vi "GTH-V2.Calibration.vi"(10 "Channel":enum16{"ChanA", "ChanB", "ChanC", "DAC"}(ring), 11 "VISA资源输入":refnum<visa-resource-name>="USB0::0x3323::0x0001::48E3845A3737::RAW") -> (0 "Error Out":errorcluster caption="错误输出", 3 "OK?":bool=TRUE)   [LabVIEW 2012, in "Lib_UEL.ATE.lvlib" / "STM32-CoreBD.lvlib"]
uses:
  STM32-CoreBD.lvlib
  <vilib>/Analysis/6fits.llb/Curve Fitting Criteria.ctl
  <vilib>/Utility/error.llb/whitespace.ctl
  <vilib>/Analysis/NI_AALPro.lvlib
panel:
  in  "Cal_DAC_Calibration":bool
  in  "Write_Data2GTH":bool
  out "Output":string[](array[string])=["\"2015-08-13,A10.032103,-65.663675\"", "\"2015-08-13,A20.012065,-24.682644\""]
  in  "Calibration Data":T1(array[cluster])=[{"ADC_Input"=1.0, "AD_Average"=5.0, "Code"="DAC"}, {"ADC_Input"=2.0, "AD_Average"=4.89, "Code"=""}, {"ADC_Input"=5.0, "AD_Average"=4.75, "Code"=""}, {"ADC_Input"=10.0, "AD_Average"=4.64, "Code"=""}, {"ADC_Input"=20.0, "AD_Average"=4.58, "Code"=""}, {"ADC_Input"=40.0, "AD_Average"=4.55, "Code"=""}, {"ADC_Input"=60.0, "AD_Average"=4.52, "Code"=""}]
  out "Best Linear Fit":dbl[][](array[numeric])=[[-3.0307985609221846, -3.030760037102811, -0.03999927599256473, -0.04186061853172174, 3.0287247066283762, 3.0301693498546984, -11.887892056086434, -11.886032639738248, 11.925863712026215, 11.928585419864591], [-3.009918735990917, -3.004162071768343, -0.02169820983103915, -0.021439537573563556, 3.0120375339021845, 3.005145559071942, -11.908703102077157, -11.899011096579235, 11.923308386282827, 11.920441274563307]] caption="最佳线性拟合"
  in  "Cal_ADC_Calibration":bool
  in  "停止":bool
  in  "RST_ADC_Value":bool
  in  "Get_ADC_Value":bool
  in  "ADC Input":dbl=11.914
  out "AD Average":dbl=3033.83968
  # "Version History\nV1.0.0, 2015-8-10, GTH-V2初始版本.\n- 每次使用前,请RST Calibration Data\n- ADC的数据是连接USB采样\n- CHAN A输入电压值: +/-3V, 0, +/-12V\n- CHAN B输入电压值: +/-1V, 0, +/-1.5V\n- CHAN C输入电压值: 1.xmA, 12.xmA\n\n- DAC数据需要手动输入.频率(Hz)幅度(mVpp)\n  1k,2k,5k,10k,20k,40k,60k\n   插上跳线帽,1k负载，1kHz，5VPP(1.76Vrms）"
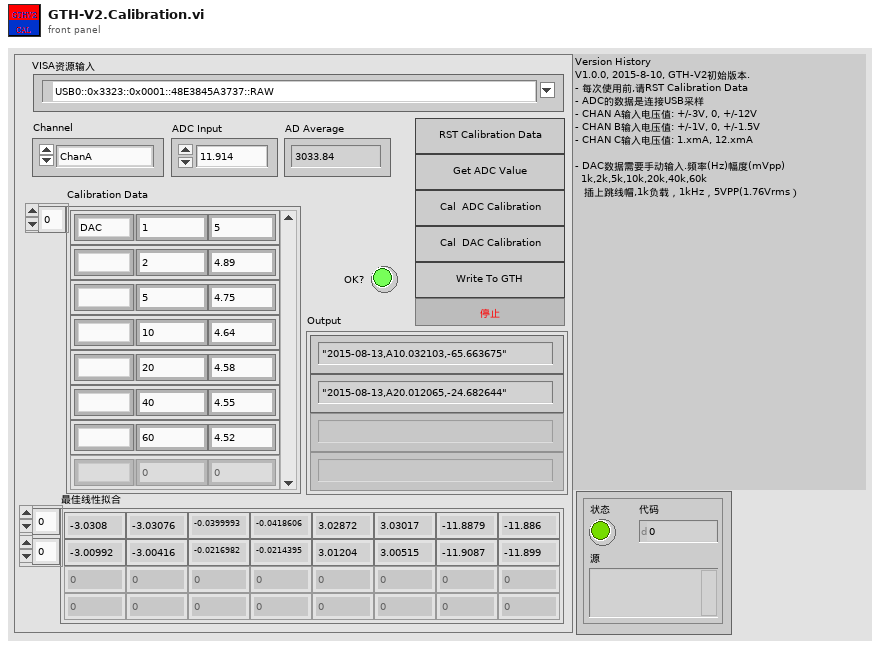
[diagram p1: front panel]
types:
  T1 = cluster{"ADC_Input":dbl, "AD_Average":dbl, "Code":string}[]
  T2 = enum16{"RelayA1", "RelayA2", "RelayA3", "RelayA4", "RelayA5", "RelayA6", "RelayA7", "RelayA8", "RelayA9", "RelayA10", "RelayB1", "RelayB2", "RelayB3", "RelayB4", "RelayB5", "RelayB6", "RelayB7", "RelayB8", "RelayB9", "RelayB10", "ADC1", "ADC2", "ADC3", "DAC1"}
  T3 = cluster{"ADC_Input":dbl, "AD_Average":dbl, "Code":string}
  T4 = enum16{"Read_Version", "Read_PID", "Read_CalibrationInfo", "Read_C_Value_ADC_ChanA", "Read_C_Value_ADC_ChanB", "Read_C_Value_Current", "Read_C_Value_DAC", "Write_CalibrationInfo", "Write_C_Value_ADC_ChanA", "Write_C_Value_ADC_ChanB", "Write_C_Value_Current", "Write_C_Value_DAC"}
  T5 = typedef "NI_AALPro.lvlib/Curve Fitting Criteria.ctl" = u16
  T6 = typedef "whitespace.ctl" = u16
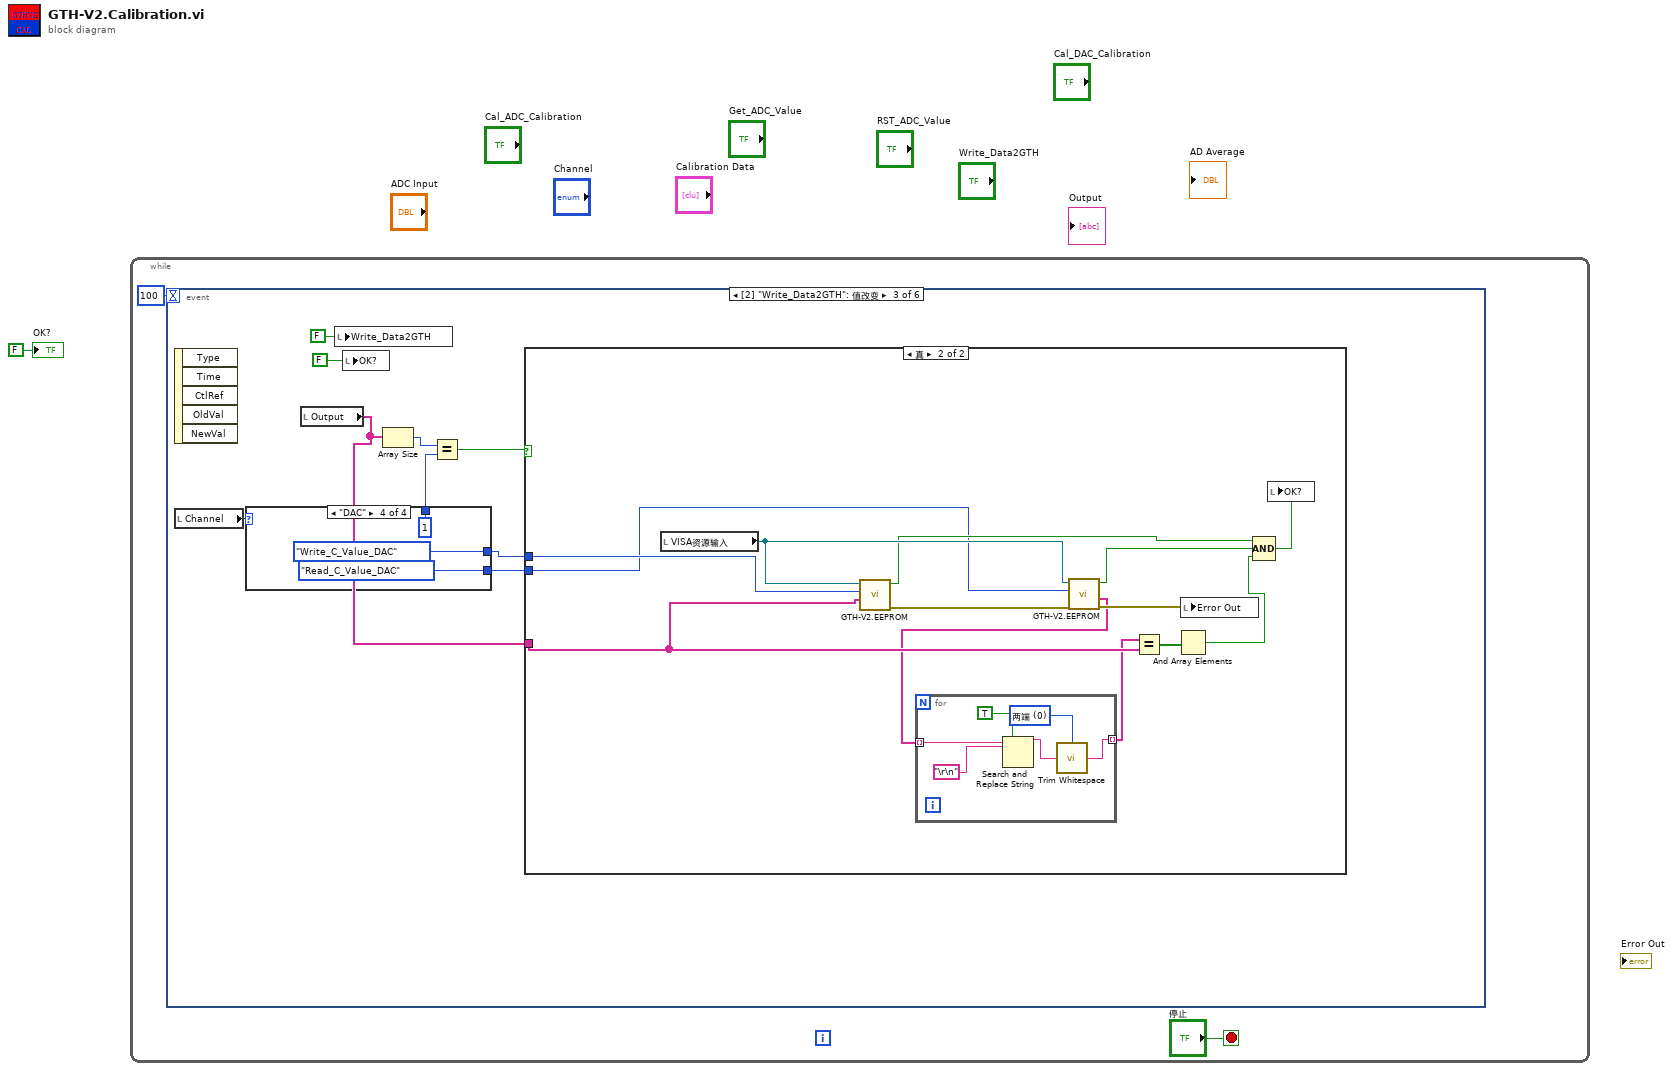
[diagram p0: block diagram]
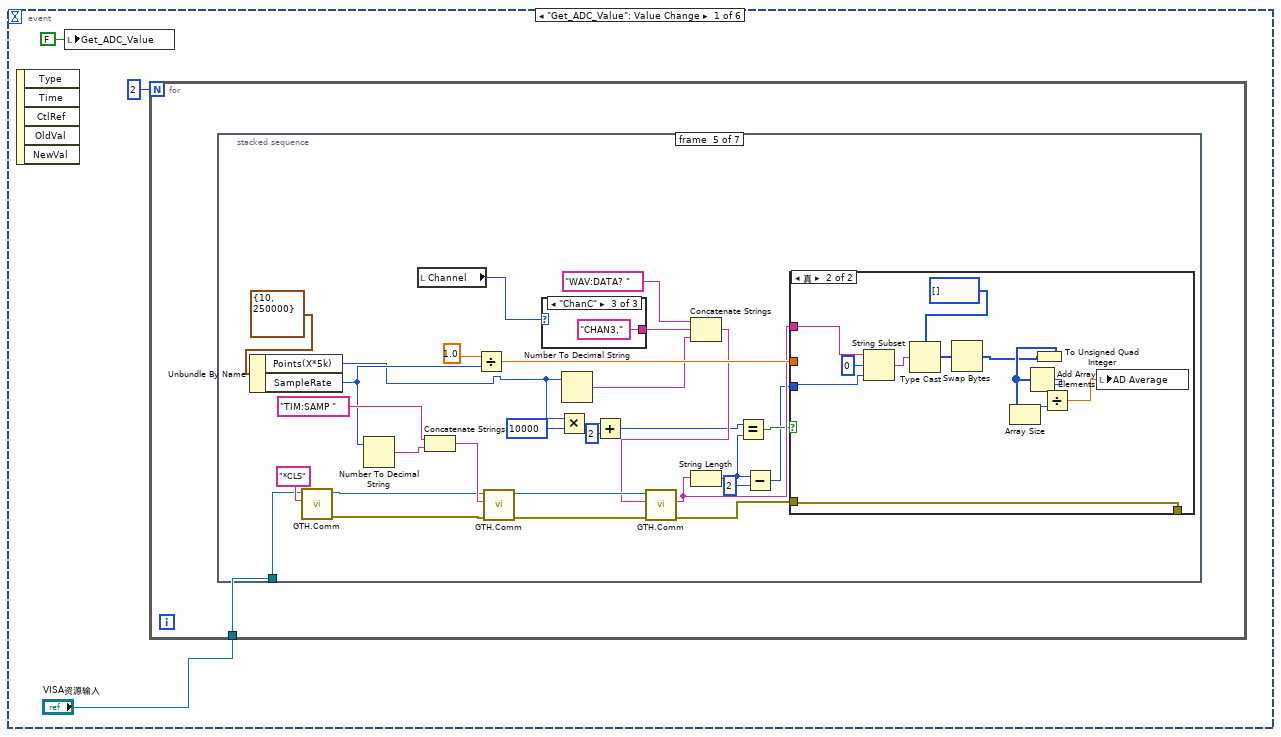
[diagram p2: hidden frame]
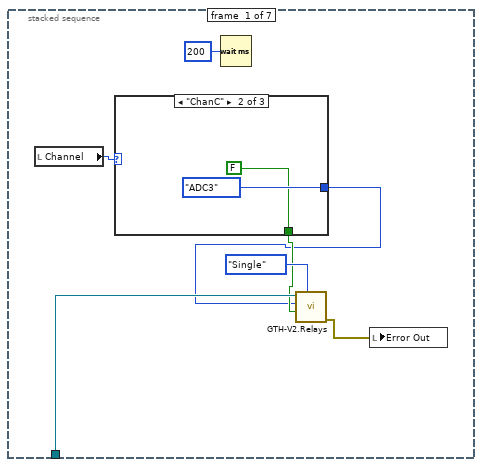
[diagram p3: hidden frame]
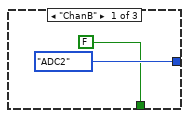
[diagram p4: hidden frame]
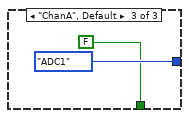
[diagram p5: hidden frame]
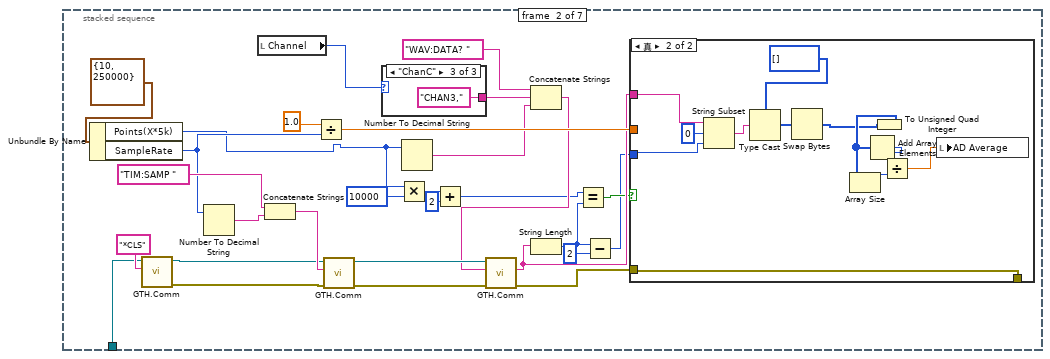
[diagram p6: hidden frame]
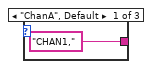
[diagram p8: hidden frame]
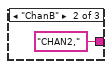
[diagram p9: hidden frame]
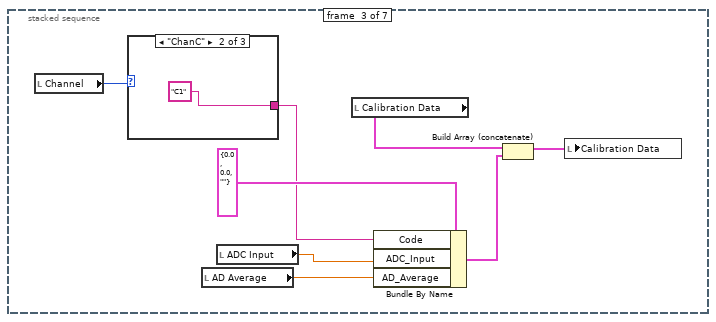
[diagram p10: hidden frame]
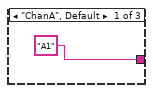
[diagram p11: hidden frame]
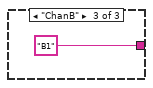
[diagram p12: hidden frame]
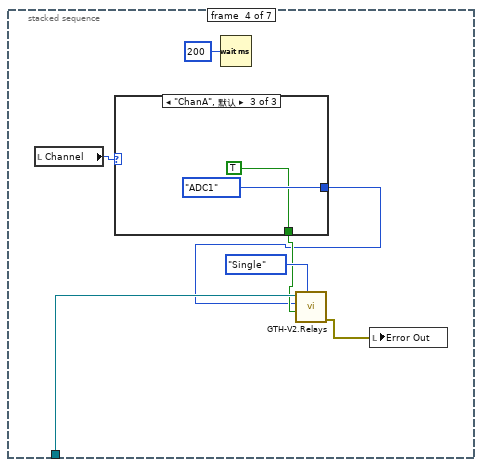
[diagram p13: hidden frame]
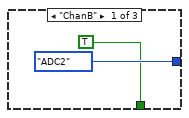
[diagram p14: hidden frame]
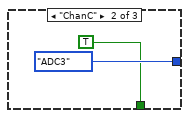
[diagram p15: hidden frame]
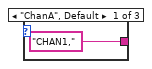
[diagram p17: hidden frame]
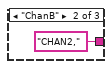
[diagram p18: hidden frame]
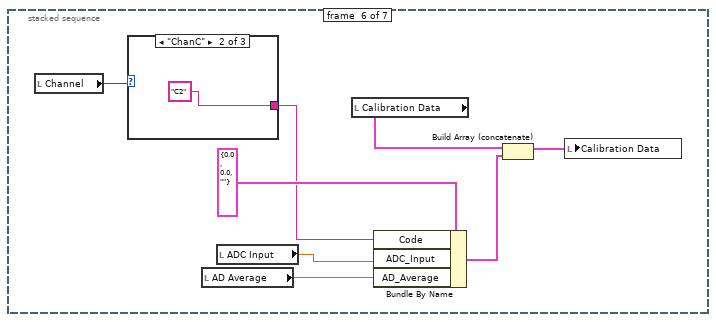
[diagram p19: hidden frame]
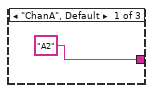
[diagram p20: hidden frame]
diagram:
  n1 = while {
    stop <- "停止" stop-if-true
    n2 = event shown="[2] \"Write_Data2GTH\": 值改变" {
      selector: _ -> [_ _ _ _ _ _]
      dyn-events: _ -> [_ _ _ _ _ _]
      timeout: 100 -> [_ _ _ _ _ _]
      event "Get_ADC_Value": Value Change {
        n3 = event-data() -> ()  [unwired: 1 in, 5 out]
        n4 = local write "Get_ADC_Value"(FALSE ("Get_ADC_Value")) -> ()
        n5 = for {
          N: 2 -> [_]
          tunnel: "VISA资源输入" -> [w7]
          n6 = stacked-sequence {
            tunnel: w7 -> [w12 w23 _ w81 w92 _ _]
            frame #0 {
              n7 = local read "Channel"() -> (w10:enum16{"ChanA", "ChanB", "ChanC", "DAC"})
              n8 = case shown="\"ChanC\"" w10 {
                tunnel: [T2."ADC2" ("Para") T2."ADC3" ("Para") T2."ADC1" ("Para")] -> w8
                tunnel: [FALSE ("ON/FF") FALSE ("ON/FF") FALSE ("ON/FF")] -> w9
                frame "ChanB" {
                }
                frame "ChanC" {
                }
                frame "ChanA", Default {
                }
              }
              n9 = Wait (ms)(milliseconds to wait=u32 200 ("等待时间（毫秒）")) -> ()  [unwired: 1 out]
              n10 = call "GTH-V2.Relays.vi"("CMD"=enum16{"All", "ChanA", "ChanB", "Single"}."Single", "ON/FF"=w9, "Para"=w8, "VISA资源输入"=w12) -> ("Error Out"=w13:errorcluster)  [unwired: 5 in, 2 out]
              n11 = local write "Error Out"(w13) -> ()
            }
            frame #1 {
              n12 = Unbundle By Name(cluster{"Points(X*5k)":u8, "SampleRate":u32} {"Points(X*5k)"=10, "SampleRate"=250000} ("ADC_Para")) -> ("Points(X*5k)"=w24:u8, "SampleRate"=w25:u32)
              n13 = call "GTH.Comm.vi"("SCPI CMD"="*CLS" ("字符串"), "USB Port In"=w23) -> ("Error Out"=w40:errorcluster, "USB Port Out"=w41:refnum<visa-resource-name>)  [unwired: 4 in, 4 out]
              n14 = Number To Decimal String(number=w25) -> (decimal integer string=w43:string)  [unwired: 1 in]
              n15 = local read "Channel"() -> (w21:enum16{"ChanA", "ChanB", "ChanC", "DAC"})
              n16 = Concatenate Strings("TIM:SAMP " ("字符串"), w43) -> (w42:string)
              n17 = Divide(x=1.0 ("y"), y=w25) -> (x/y=w46:dbl)
              n18 = call "GTH.Comm.vi"("Error In"=w40, "SCPI CMD"=w42, "USB Port In"=w41) -> ("Error Out"=w37:errorcluster, "USB Port Out"=w38:refnum<visa-resource-name>)  [unwired: 3 in, 4 out]
              n19 = case shown="\"ChanC\"" w21 {
                tunnel: ["CHAN1," ("字符串") "CHAN2," ("字符串") "CHAN3," ("字符串")] -> w48
                frame "ChanA", Default {
                }
                frame "ChanB" {
                }
                frame "ChanC" {
                }
              }
              n20 = Multiply(x=w24, y=u32 10000) -> (x*y=w33:u32)
              n21 = Number To Decimal String(number=w24) -> (decimal integer string=w39:string)  [unwired: 1 in]
              n22 = Add(x=w33, y=u32 2) -> (x+y=w30:u32)
              n23 = Concatenate Strings("WAV:DATA? " ("字符串"), w48, w39) -> (w36:string)
              n24 = call "GTH.Comm.vi"("Error In"=w37, "SCPI CMD"=w36, "USB Port In"=w38) -> ("Error Out"=w35:errorcluster, "Return"=w31:string)  [unwired: 3 in, 4 out]
              n25 = String Length(string=w31) -> (length=w28:i32)
              n26 = Equal?(x=w30, y=w28) -> (x = y?=w29:bool)
              n27 = Subtract(x=w28, y=2) -> (x-y=w26:i32)
              n28 = case shown="真" w29 {
                tunnel: w46 -> [_ _]
                tunnel: [w50 w52] -> _
                tunnel: w35 -> [w50 w52]
                tunnel: w31 -> [_ w59]
                tunnel: w26 -> [_ w57]
                frame False {
                }
                frame True {
                  n29 = String Subset(string=w59, offset (0)=0 ("偏移量(0)"), length (rest)=w57) -> (substring=w60:string)
                  n30 = Type Cast(type=u16[] [], x=w60) -> (*(type *) &x=w61:u16[])
                  n31 = Swap Bytes(anything=w61) -> (byte swapped=w53:u16[])
                  n32 = To Unsigned Quad Integer(1:w53) -> (0:w54:u64[])
                  n33 = Array Size(array=w54) -> (size(s)=w55:i32)
                  n34 = Add Array Elements(numeric array=w54) -> (sum=w56:u64)
                  n35 = Divide(x=w56, y=w55) -> (x/y=w51:dbl)
                  n36 = local write "AD Average"(w51) -> ()
                }
              }
            }
            frame #2 {
              n37 = local read "Channel"() -> (w66:enum16{"ChanA", "ChanB", "ChanC", "DAC"})
              n38 = case shown="\"ChanC\"" w66 {
                tunnel: ["A1" ("Code") "C1" ("Code") "B1" ("Code")] -> w67
                frame "ChanA", Default {
                }
                frame "ChanC" {
                }
                frame "ChanB" {
                }
              }
              n39 = local read "AD Average"() -> (w72:dbl)
              n40 = local read "ADC Input"() -> (w71:dbl)
              n41 = local read "Calibration Data"() -> (w70:T1)
              n42 = Bundle By Name(cluster=T3 {"ADC_Input"=0.0, "AD_Average"=0.0, "Code"=""} ("簇"), "Code"=w67, "ADC_Input"=w71, "AD_Average"=w72) -> (w69:T3)
              n43 = Build Array (concatenate)(w70, w69) -> (w68:T1)
              n44 = local write "Calibration Data"(w68) -> ()
            }
            frame #3 {
              n45 = local read "Channel"() -> (w79:enum16{"ChanA", "ChanB", "ChanC", "DAC"})
              n46 = case shown="\"ChanA\", 默认" w79 {
                tunnel: [T2."ADC2" ("Para") T2."ADC3" ("Para") T2."ADC1" ("Para")] -> w77
                tunnel: [TRUE ("ON/FF") TRUE ("ON/FF") TRUE ("ON/FF")] -> w78
                frame "ChanB" {
                }
                frame "ChanC" {
                }
                frame "ChanA", Default {
                }
              }
              n47 = Wait (ms)(milliseconds to wait=u32 200 ("等待时间（毫秒）")) -> ()  [unwired: 1 out]
              n48 = call "GTH-V2.Relays.vi"("CMD"=enum16{"All", "ChanA", "ChanB", "Single"}."Single", "ON/FF"=w78, "Para"=w77, "VISA资源输入"=w81) -> ("Error Out"=w82:errorcluster)  [unwired: 5 in, 2 out]
              n49 = local write "Error Out"(w82) -> ()
            }
            frame #4 {
              n50 = Unbundle By Name(cluster{"Points(X*5k)":u8, "SampleRate":u32} {"Points(X*5k)"=10, "SampleRate"=250000} ("ADC_Para")) -> ("Points(X*5k)"=w93:u8, "SampleRate"=w94:u32)
              n51 = call "GTH.Comm.vi"("SCPI CMD"="*CLS" ("字符串"), "USB Port In"=w92) -> ("Error Out"=w109:errorcluster, "USB Port Out"=w110:refnum<visa-resource-name>)  [unwired: 4 in, 4 out]
              n52 = Number To Decimal String(number=w94) -> (decimal integer string=w112:string)  [unwired: 1 in]
              n53 = local read "Channel"() -> (w90:enum16{"ChanA", "ChanB", "ChanC", "DAC"})
              n54 = Concatenate Strings("TIM:SAMP " ("字符串"), w112) -> (w111:string)
              n55 = Divide(x=1.0 ("y"), y=w94) -> (x/y=w115:dbl)
              n56 = call "GTH.Comm.vi"("Error In"=w109, "SCPI CMD"=w111, "USB Port In"=w110) -> ("Error Out"=w106:errorcluster, "USB Port Out"=w107:refnum<visa-resource-name>)  [unwired: 3 in, 4 out]
              n57 = case shown="\"ChanC\"" w90 {
                tunnel: ["CHAN1," ("字符串") "CHAN2," ("字符串") "CHAN3," ("字符串")] -> w117
                frame "ChanA", Default {
                }
                frame "ChanB" {
                }
                frame "ChanC" {
                }
              }
              n58 = Multiply(x=w93, y=u32 10000) -> (x*y=w102:u32)
              n59 = Number To Decimal String(number=w93) -> (decimal integer string=w108:string)  [unwired: 1 in]
              n60 = Add(x=w102, y=u32 2) -> (x+y=w99:u32)
              n61 = Concatenate Strings("WAV:DATA? " ("字符串"), w117, w108) -> (w105:string)
              n62 = call "GTH.Comm.vi"("Error In"=w106, "SCPI CMD"=w105, "USB Port In"=w107) -> ("Error Out"=w104:errorcluster, "Return"=w100:string)  [unwired: 3 in, 4 out]
              n63 = String Length(string=w100) -> (length=w97:i32)
              n64 = Equal?(x=w99, y=w97) -> (x = y?=w98:bool)
              n65 = Subtract(x=w97, y=2) -> (x-y=w95:i32)
              n66 = case shown="真" w98 {
                tunnel: w115 -> [_ _]
                tunnel: [w119 w121] -> _
                tunnel: w104 -> [w119 w121]
                tunnel: w100 -> [_ w128]
                tunnel: w95 -> [_ w126]
                frame False {
                }
                frame True {
                  n67 = String Subset(string=w128, offset (0)=0 ("偏移量(0)"), length (rest)=w126) -> (substring=w129:string)
                  n68 = Type Cast(type=u16[] [], x=w129) -> (*(type *) &x=w130:u16[])
                  n69 = Swap Bytes(anything=w130) -> (byte swapped=w122:u16[])
                  n70 = To Unsigned Quad Integer(1:w122) -> (0:w123:u64[])
                  n71 = Array Size(array=w123) -> (size(s)=w124:i32)
                  n72 = Add Array Elements(numeric array=w123) -> (sum=w125:u64)
                  n73 = Divide(x=w125, y=w124) -> (x/y=w120:dbl)
                  n74 = local write "AD Average"(w120) -> ()
                }
              }
            }
            frame #5 {
              n75 = local read "Channel"() -> (w135:enum16{"ChanA", "ChanB", "ChanC", "DAC"})
              n76 = case shown="\"ChanC\"" w135 {
                tunnel: ["A2" ("Code") "C2" ("Code") "B2" ("Code")] -> w136
                frame "ChanA", Default {
                }
                frame "ChanC" {
                }
                frame "ChanB" {
                }
              }
              n77 = local read "AD Average"() -> (w141:dbl)
              n78 = local read "ADC Input"() -> (w140:dbl)
              n79 = local read "Calibration Data"() -> (w139:T1)
              n80 = Bundle By Name(cluster=T3 {"ADC_Input"=0.0, "AD_Average"=0.0, "Code"=""} ("簇"), "Code"=w136, "ADC_Input"=w140, "AD_Average"=w141) -> (w138:T3)
              n81 = Build Array (concatenate)(w139, w138) -> (w137:T1)
              n82 = local write "Calibration Data"(w137) -> ()
            }
            frame #6 {
              n83 = Wait (ms)(milliseconds to wait=u32 500 ("等待时间（毫秒）")) -> ()  [unwired: 1 out]
            }
          }
        }
      }
      event "Cal_DAC_Calibration": Value Change {
        n84 = event-data() -> ()  [unwired: 1 in, 5 out]
        n85 = local read "Calibration Data"() -> (w150:T1)
        n86 = local write "Cal_DAC_Calibration"(FALSE ("Cal_DAC_Calibration")) -> ()
        n87 = Array Size(array=w150) -> (size(s)=w149:i32)
        n88 = Greater Or Equal?(x=w149, y=6) -> (x >= y?=w147:bool)
        n89 = case shown="真" w147 {
          tunnel: w150 -> [_ w170]
          frame False {
          }
          frame True {
            w160 = "," ("时间格式字符串(%c)")
            w169 = T5 0 items=["最小二乘", "最小绝对残差", "Bisquare"] ("method")
            w171 = dbl[] []
            n90 = for {
              tunnel: w170 -> [w178] mode=indexing
              shift-right: [w176] -> w153
              shift-left: w171 -> [w173]
              shift-right: [w175] -> w154
              shift-left: w171 -> [w172]
              n91 = Unbundle By Name(w178) -> ("ADC_Input"=w177:dbl, "AD_Average"=w174:dbl)
              n92 = Build Array (concatenate)(w173, w177) -> (w176:dbl[])
              n93 = Build Array (concatenate)(w172, w174) -> (w175:dbl[])
            }
            n94 = Get Date/Time In Seconds() -> (seconds since 1Jan1904=w164:timestamp)
            n95 = Format Date/Time String(time format string (%c)="%Y-%m-%d" ("时间格式字符串(%c)"), seconds (now)=w164) -> (date/time string=w162:string)  [unwired: 1 in]
            n96 = call <vilib>:"Power Fit.vi"("Y"=w154, "X"=w153, "method"=w169) -> ("Best Power Fit"=w167:dbl[], "amplitude"=w158:dbl, "power"=w157:dbl, "offset"=w156:dbl)  [unwired: 7 in, 2 out]
            n97 = Number To Fractional String(number=w158) -> (F-format string=w165:string)  [unwired: 3 in]
            n98 = Number To Fractional String(number=w157) -> (F-format string=w166:string)  [unwired: 3 in]
            n99 = Number To Fractional String(number=w156) -> (F-format string=w159:string)  [unwired: 3 in]
            n100 = Build Array(w167) -> (w168:dbl[][])
            n101 = local write "Best Linear Fit"(w168) -> ()
            n102 = Concatenate Strings(w162, w160, "DAC" ("字符串"), w160, w165, w160, w166, w160, w159) -> (w152:string)
            n103 = Build Array(w152) -> (w155:string[])
            n104 = local write "Output"(w155) -> ()
          }
        }
      }
      event "Write_Data2GTH": Value Change {
        n105 = event-data() -> ()  [unwired: 1 in, 5 out]
        n106 = local read "Channel"() -> (w182:enum16{"ChanA", "ChanB", "ChanC", "DAC"})
        n107 = case shown="\"DAC\"" w182 {
          tunnel: [T4."Write_C_Value_ADC_ChanB" ("CMD") T4."Write_C_Value_Current" ("CMD") T4."Write_C_Value_ADC_ChanA" ("CMD") T4."Write_C_Value_DAC" ("CMD")] -> w181
          tunnel: [T4."Read_C_Value_ADC_ChanB" ("CMD") T4."Read_C_Value_Current" ("CMD") T4."Read_C_Value_ADC_ChanA" ("CMD") T4."Read_C_Value_DAC" ("CMD")] -> w180
          tunnel: [2 ("y") 2 ("y") 2 ("y") 1 ("y")] -> w179
          frame "ChanB" {
          }
          frame "ChanC" {
          }
          frame "ChanA" {
          }
          frame "DAC" {
          }
        }
        n108 = local read "Output"() -> (w183:string[])
        n109 = local write "Write_Data2GTH"(FALSE ("Write_Data2GTH")) -> ()
        n110 = local write "OK?"(FALSE ("OK?")) -> ()
        n111 = Array Size(array=w183) -> (size(s)=w185:i32)
        n112 = Equal?(x=w185, y=w179) -> (x = y?=w184:bool)
        n113 = case shown="真" w184 {
          tunnel: w183 -> [_ w210]
          tunnel: w181 -> [_ w201]
          tunnel: w180 -> [_ w200]
          frame False {
          }
          frame True {
            n114 = local read "VISA资源输入"() -> (w212:refnum<visa-resource-name>)
            n115 = call "GTH-V2.EEPROM.vi"("Calibration_Value_In"=w210, "CMD"=w201, "VISA资源输入"=w212) -> ("Error Out"=w211:errorcluster, "OK?"=w205:bool)  [unwired: 6 in, 1 out]
            n116 = call "GTH-V2.EEPROM.vi"("Error In"=w211, "CMD"=w200, "VISA资源输入"=w212) -> ("Error Out"=w208:errorcluster, "Calibration_Value_Out"=w203:string[], "OK?"=w206:bool)  [unwired: 6 in]
            n117 = for {
              tunnel: w203 -> [w218] mode=indexing
              tunnel: [w214] -> w202 mode=indexing
              w213 = T6 0 items=["两端", "字符串首端", "字符串末端"] ("location (both)")
              n118 = Search and Replace String(replace all?=TRUE ("替换全部？(F)"), input string=w218, search string="\r\n") -> (result string=w215:string)  [unwired: 5 in, 3 out]
              n119 = call <vilib>:"Trim Whitespace.vi"("string"=w215, "location (both)"=w213) -> ("trimmed string"=w214:string)
            }
            n120 = Equal?(x=w202, y=w210) -> (x = y?=w209:bool[])
            n121 = And Array Elements(Boolean array=w209) -> (logical AND=w207:bool)
            n122 = local write "Error Out"(w208) -> ()
            n123 = Compound Arithmetic op=AND(w205, w206, w207) -> (w204:bool)
            n124 = local write "OK?"(w204) -> ()
          }
        }
      }
      event "RST_ADC_Value": Value Change {
        n125 = event-data() -> ()  [unwired: 1 in, 5 out]
        n126 = local write "Calibration Data"(T1 [] ("Calibration Data")) -> ()
        n127 = local write "RST_ADC_Value"(FALSE ("RST_ADC_Value")) -> ()
        n128 = local write "Output"(string[] [] ("Output")) -> ()
      }
      event "Cal_ADC_Calibration": Value Change {
        n129 = event-data() -> ()  [unwired: 1 in, 5 out]
        n130 = local write "Cal_ADC_Calibration"(FALSE ("Cal_ADC_Calibration")) -> ()
        n131 = stacked-sequence {
          seq-local: [w225 _] -> [_ w282]
          seq-local: [w226 _] -> [_ w283]
          seq-local: [w224 _] -> [_ w280]
          seq-local: [w223 _] -> [_ w279]
          frame #0 {
            w227 = dbl[] []
            n132 = local read "Calibration Data"() -> (w228:T1)
            n133 = for {
              tunnel: w228 -> [w244] mode=indexing
              shift-right: [w242] -> w226
              shift-left: w227 -> [w234]
              shift-right: [w241] -> w225
              shift-left: w227 -> [w233]
              shift-right: [w232] -> w224
              shift-left: w227 -> [w231]
              shift-right: [w230] -> w223
              shift-left: w227 -> [w229]
              n134 = Unbundle By Name(w244) -> ("Code"=w239:string, "ADC_Input"=w243:dbl, "AD_Average"=w240:dbl)
              n135 = Decimal String To Number(string=w239, offset=1 ("偏移量")) -> (number=w237:i32)  [unwired: 1 in, 1 out]
              n136 = Equal?(x=w237, y=1) -> (x = y?=w235:bool)
              n137 = case shown="真" w235 {
                tunnel: w243 -> [w247 w260]
                tunnel: [w252 w259] -> w242
                tunnel: [w251 w258] -> w241
                tunnel: w240 -> [w246 w257]
                tunnel: w234 -> [w252 w256]
                tunnel: w233 -> [w251 w255]
                tunnel: [w250 w254] -> w232
                tunnel: w231 -> [w249 w254]
                tunnel: [w245 w253] -> w230
                tunnel: w229 -> [w248 w253]
                frame False {
                  n138 = Build Array (concatenate)(w249, w247) -> (w250:dbl[])
                  n139 = Build Array (concatenate)(w248, w246) -> (w245:dbl[])
                }
                frame True {
                  n140 = Build Array (concatenate)(w256, w260) -> (w259:dbl[])
                  n141 = Build Array (concatenate)(w255, w257) -> (w258:dbl[])
                }
              }
            }
          }
          frame #1 {
            w265 = "," ("时间格式字符串(%c)")
            w262 = "," ("时间格式字符串(%c)")
            w278 = T5 0 items=["最小二乘", "最小绝对残差", "Bisquare"] ("method")
            n142 = Get Date/Time In Seconds() -> (seconds since 1Jan1904=w287:timestamp)
            n143 = local read "Channel"() -> (w272:enum16{"ChanA", "ChanB", "ChanC", "DAC"})
            n144 = Format Date/Time String(time format string (%c)="%Y-%m-%d," ("时间格式字符串(%c)"), seconds (now)=w287) -> (date/time string=w273:string)  [unwired: 1 in]
            n145 = case shown="\"ChanA\", 默认" w272 {
              tunnel: ["B1" ("时间格式字符串(%c)") "A1" ("时间格式字符串(%c)") "C1" ("时间格式字符串(%c)")] -> w271
              tunnel: ["B2" ("时间格式字符串(%c)") "A2" ("时间格式字符串(%c)") "C2" ("时间格式字符串(%c)")] -> w270
              frame "ChanB" {
              }
              frame "ChanA", Default {
              }
              frame "ChanC" {
              }
            }
            n146 = call <vilib>:"Linear Fit.vi"("Y"=w283, "X"=w282, "method"=w278) -> ("Best Linear Fit"=w281:dbl[], "slope"=w285:dbl, "intercept"=w284:dbl)  [unwired: 8 in, 2 out]
            n147 = call <vilib>:"Linear Fit.vi"("Y"=w280, "X"=w279, "method"=w278) -> ("Best Linear Fit"=w277:dbl[], "slope"=w275:dbl, "intercept"=w274:dbl)  [unwired: 8 in, 2 out]
            n148 = Number To Fractional String(number=w285) -> (F-format string=w263:string)  [unwired: 3 in]
            n149 = Number To Fractional String(number=w284) -> (F-format string=w264:string)  [unwired: 3 in]
            n150 = Number To Fractional String(number=w275) -> (F-format string=w266:string)  [unwired: 3 in]
            n151 = Number To Fractional String(number=w274) -> (F-format string=w267:string)  [unwired: 3 in]
            n152 = Build Array(w281, w277) -> (→"Best Linear Fit":dbl[][])
            n153 = Concatenate Strings(w273, w271, w262, w263, w262, w264) -> (w269:string)
            n154 = Concatenate Strings(w273, w270, w265, w266, w265, w267) -> (w268:string)
            n155 = Build Array(w269, w268) -> (w261:string[])
            n156 = local write "Output"(w261) -> ()
          }
        }
      }
      event Timeout {
        n157 = event-data() -> ()  [unwired: 1 in, 2 out]
      }
    }
  }
  "OK?" <- FALSE ("OK?")
